vi "find_fish_position_v10.vi"() -> ()   [LabVIEW 2014]
uses:
  labview/find_fish_position.lvlib
  find_fish_position_dll/Release/find_fish_position_dll.dll
panel:
  in  "Counting threshold":i32=205
  in  "background":path
  out "Centroid in":cluster{"x":i32, "y":i32}
  out "fish found":bool
  in  "Image":path
  in  "stop":bool
  out "Image":T1(plugin-control)
  out "Elapsed Time (msec)":dbl format="%0.3f"
  out "# of Trials":i32=10
  in  "shift":i32=10
  in  "ROI height":i32=256
  in  "ROI width":i32=256
  in  "setROI":bool
  in  "Esize (open)":i32(slide)=4 scale=3.0..10.0
  out "Centroid":cluster{"x":i32, "y":i32}
  in  "Esize (close)":i32(slide)=4 scale=3.0..10.0
  in  "Image Threshold":i32(slide)=205 scale=50.0..255.0
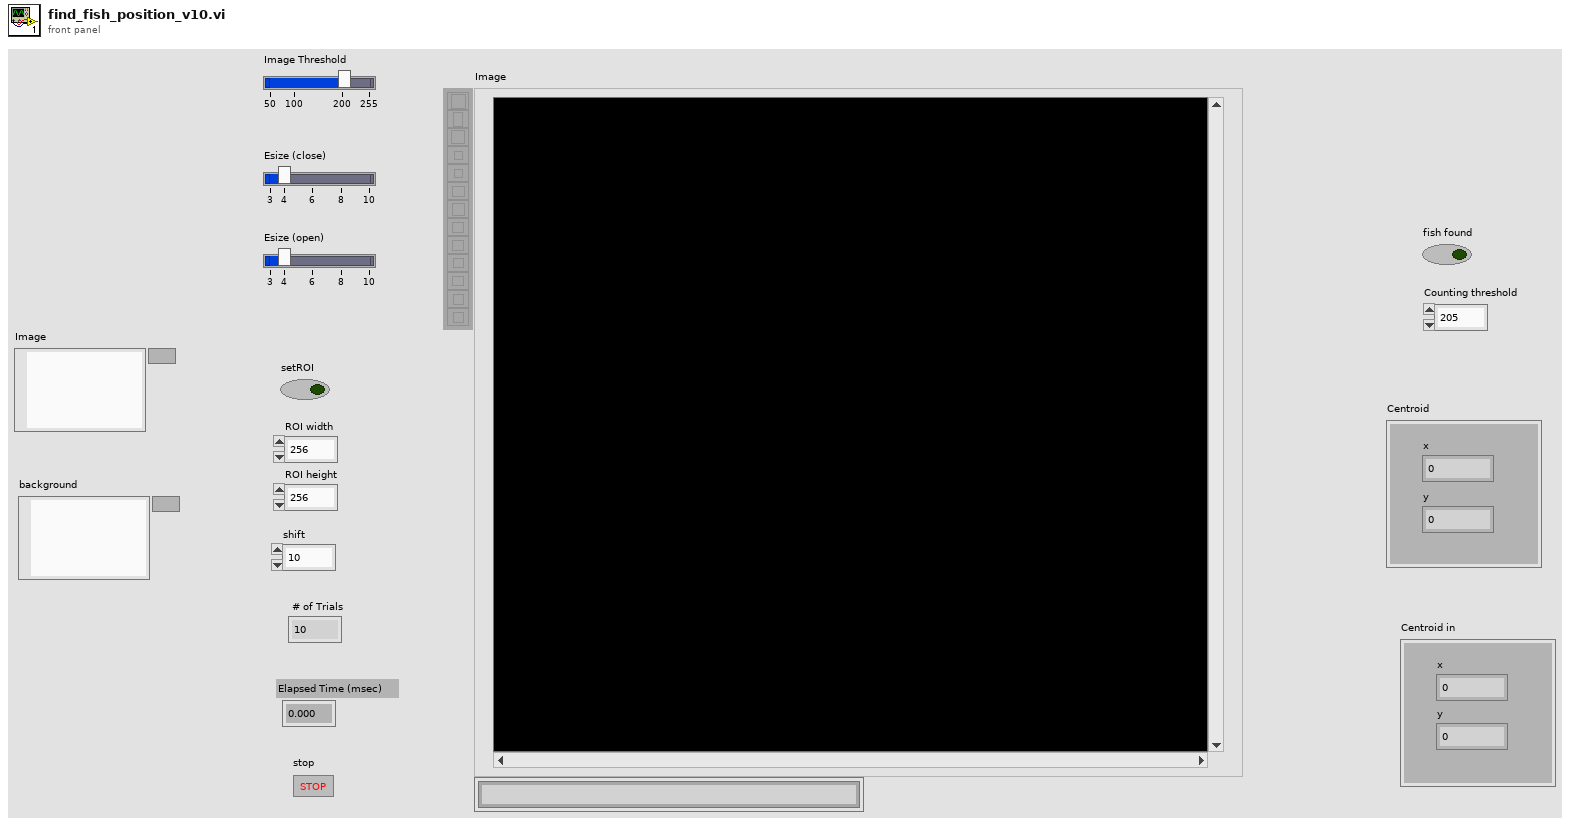
[diagram p1: front panel]
types:
  T1 = typedef "IMAQ Image.ctl" = refnum<image>
  T2 = enum32{"Map Pixel Pointer", "Unmap Pixel Pointer", "Get Pixels Infos"}
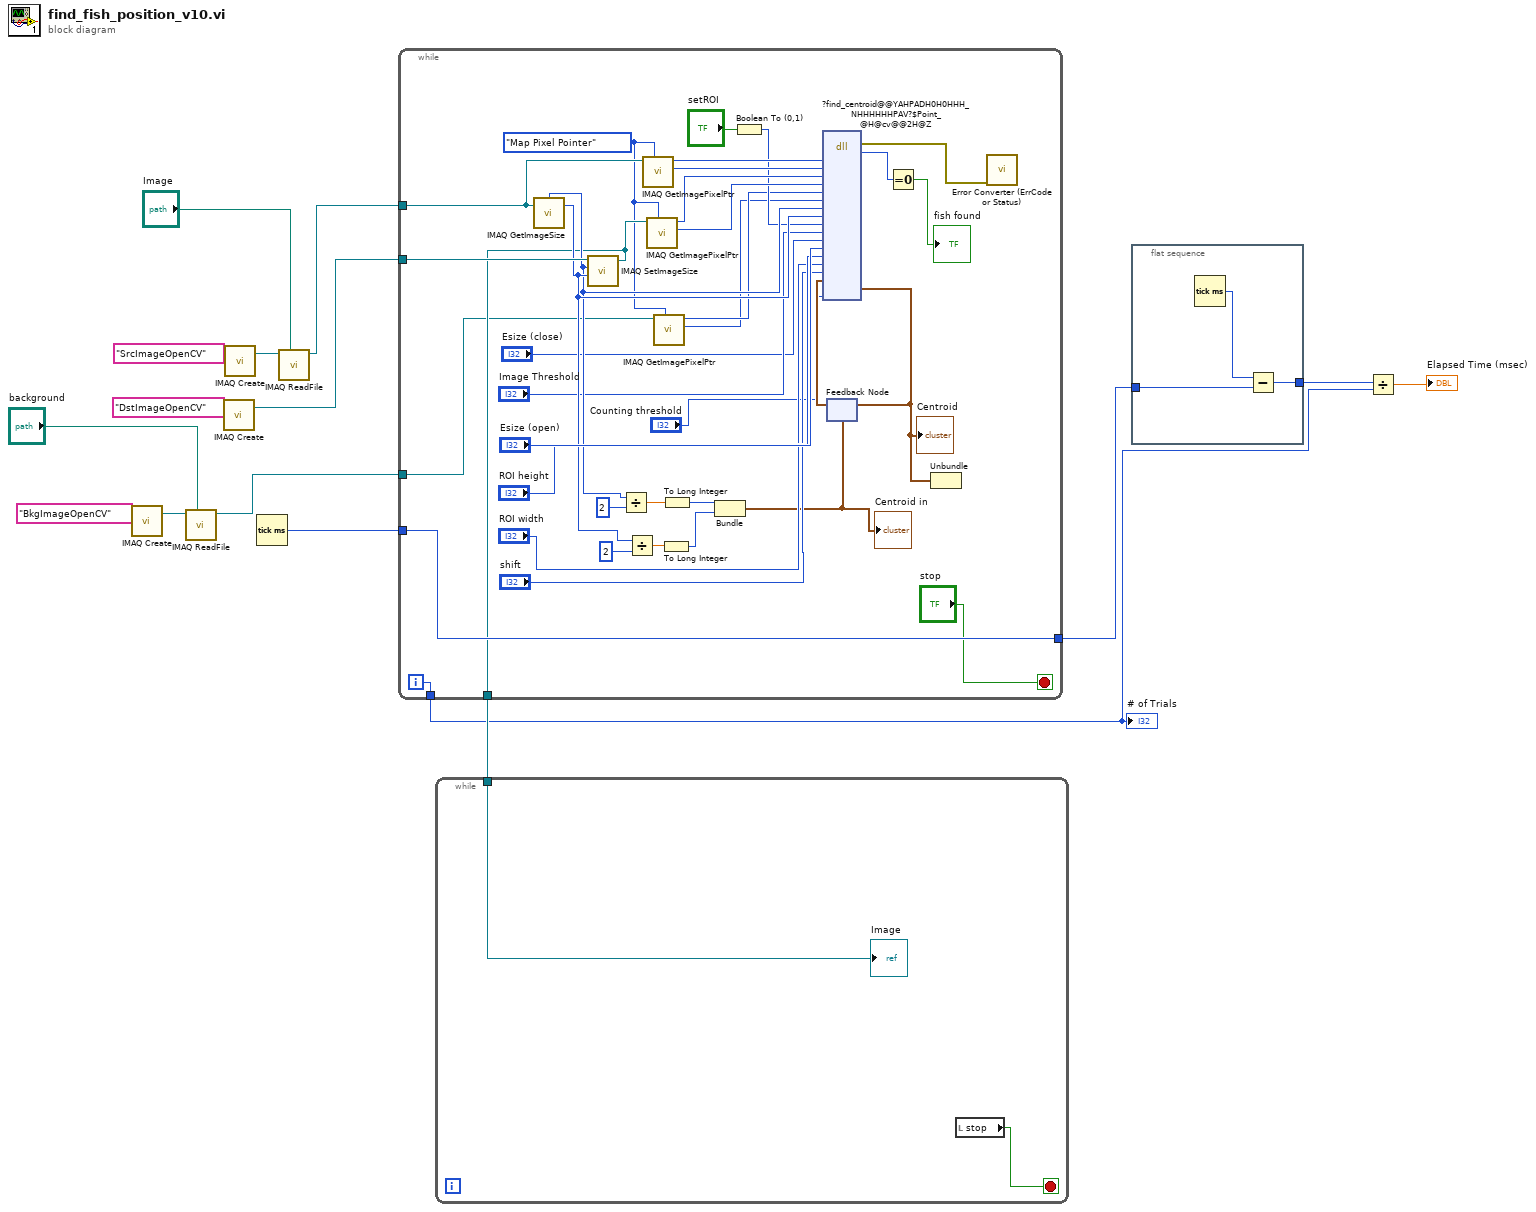
[diagram p0: block diagram]
diagram:
  n1 = call "IMAQ Create"("Image Name"="BkgImageOpenCV") -> ("New Image"=w3:T1)  [unwired: 4 in, 1 out]
  n2 = call "IMAQ ReadFile"("File Path"="background", "Image"=w3) -> ("Image Out"=w1:T1)  [unwired: 5 in, 4 out]
  n3 = call "IMAQ Create"("Image Name"="DstImageOpenCV") -> ("New Image"=w15:T1)  [unwired: 4 in, 1 out]
  n4 = call "IMAQ Create"("Image Name"="SrcImageOpenCV") -> ("New Image"=w12:T1)  [unwired: 4 in, 1 out]
  n5 = Tick Count (ms)() -> (millisecond timer value=w10:u32)
  n6 = call "IMAQ ReadFile"("File Path"="Image", "Image"=w12) -> ("Image Out"=w16:T1)  [unwired: 5 in, 4 out]
  n7 = while {
    tunnel: w16 -> [w53]
    tunnel: w15 -> [w52]
    tunnel: [w30] -> w11
    tunnel: w10 -> [w30]
    tunnel: [w29] -> w7
    tunnel: [w27] -> w6
    tunnel: w1 -> [w20]
    i -> [w27]
    stop <- "stop" stop-if-true
    w21 = T2."Map Pixel Pointer" ("Function")
    n8 = call "IMAQ GetImageSize"("Image"=w53) -> ("Y Resolution"=w50:i32, "X Resolution"=w48:i32)  [unwired: 3 in, 1 out]
    n9 = call "IMAQ SetImageSize"("Y Resolution"=w50, "X Resolution"=w48, "Image"=w52) -> ("Image Out"=w29:T1)  [unwired: 2 in, 1 out]
    n10 = Divide(x=w48, y=2) -> (x/y=w37:dbl)
    n11 = Divide(x=w50, y=2) -> (x/y=w35:dbl)
    n12 = call "IMAQ GetImagePixelPtr"("Function"=w21, "Image"=w53) -> ("LineWidth(Pixels)"=w41:i32, "Pixel Pointer out"=w40:u64)  [unwired: 4 in, 4 out]
    n13 = call "IMAQ GetImagePixelPtr"("Function"=w21, "Image"=w29) -> ("LineWidth(Pixels)"=w43:i32, "Pixel Pointer out"=w42:u64)  [unwired: 4 in, 4 out]
    n14 = call "IMAQ GetImagePixelPtr"("Function"=w21, "Image"=w20) -> ("LineWidth(Pixels)"=w18:i32, "Pixel Pointer out"=w19:u64)  [unwired: 4 in, 4 out]
    n15 = To Long Integer(number=w35) -> (32bit integer=w34:i32)
    n16 = To Long Integer(number=w37) -> (32bit integer=w36:i32)
    n17 = Bundle(w36, w34) -> (w24:cluster{i32, i32})  [unwired: 1 in]
    "Centroid in" <- w24
    n18 = Boolean To (0,1)(Boolean="setROI") -> (0, 1=w38:i16)
    n19 = feedback #1(w24) -> (w22:cluster{i32, i32})
    n20 = dll-call lib="E:/quan/fish tracking dll vc10 opencv3/find_fish_position_dll/Release/find_fish_position_dll.dll" fn="?find_centroid@@YAHPADH0H0HHH_NHHHHHHPAV?$Point_@H@cv@@2H@Z"("ImagePtrSrc"=w40, "LineWidthSrc"=w41, "ImagePtrDst"=w42, "LineWidthDst"=w43, "ImagePtrBkg"=w19, "LineWidthBkg"=w18, "Width"=w48, "Height"=w50, "setROI"=w38, "BinThreshold"="Image Threshold", "Esize_close"="Esize (close)", "Esize_open"="Esize (open)", "ROI_width"="ROI height", "ROI_height"="ROI width", "shift"="shift", "centroid_in"=w22, "counting_threshold"="Counting threshold") -> (error out=w46:errorcluster, "return type"=w26:i32, "Centroid"=w23:cluster{"x":i32, "y":i32})  [unwired: 21 in, 1 out]
    "Centroid" <- w23
    n21 = feedback-in #1(w23) -> ()
    n22 = Equal To 0?(x=w26) -> (x = 0?=→"fish found":bool)
    n23 = Unbundle(w23) -> ()  [unwired: 2 out]
    n24 = call "Error Converter (ErrCode or Status).vi"("error in (no error)"=w46) -> ()  [unwired: 10 in, 1 out]
  }
  "# of Trials" <- w6
  n25 = while {
    tunnel: w7 -> [w55]
    stop <- w54 stop-if-true
    n26 = local read "stop"() -> (w54:bool)
    "Image" <- w55
  }
  n27 = flat-sequence {
    tunnel: w11 -> [w58]
    tunnel: [w56] -> w9
    frame #0 {
      n28 = Tick Count (ms)() -> (millisecond timer value=w57:u32)
      n29 = Subtract(x=w57, y=w58) -> (x-y=w56:u32)
    }
  }
  n30 = Divide(x=w9, y=w6) -> (x/y=→"Elapsed Time (msec)":dbl)
